vi "VirtualBench_Current_Measurement_Verdict.vi"(8 "Maximum Value":dbl, 9 "Minimum Value":dbl, 11 "Measured Current":dbl) -> (3 "Pass/Fail":bool)   [LabVIEW 2016]
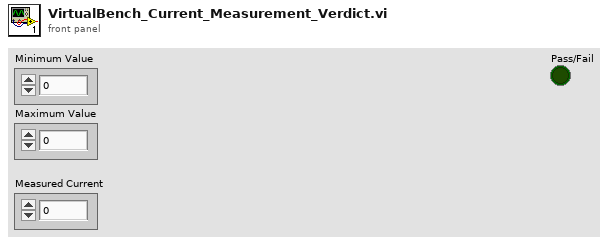
[diagram p1: front panel]
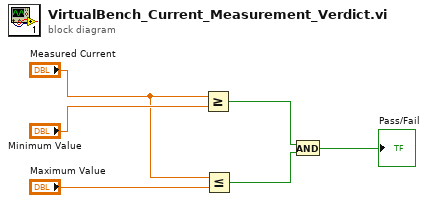
[diagram p0: block diagram]
diagram:
  n1 = Greater Or Equal?(x="Measured Current", y="Minimum Value") -> (x >= y?=w3:bool)
  n2 = Less Or Equal?(x="Measured Current", y="Maximum Value") -> (x <= y?=w2:bool)
  n3 = And(x=w3, y=w2) -> (x .and. y?=→"Pass/Fail":bool)
